vi "Enum from Ring String.vi"(8 "String to Match":string, 9 "Ring Strings []":string[](array[string]), 11 "Ring StringsAndValues[]":T1) -> (0 "error out":errorcluster, 3 "Enum Value":i32)   [LabVIEW 2023]
uses:
  <vilib>/Utility/miscctls.llb/LVStringsAndValuesArrayTypeDef_I32.ctl
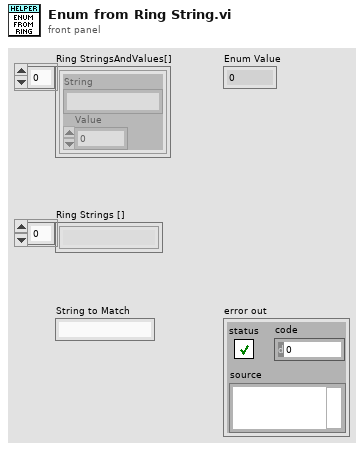
[diagram p1: front panel]
types:
  T1 = typedef "LVStringsAndValuesArrayTypeDef_I32.ctl" = cluster{"String":string, "Value":i32}[]
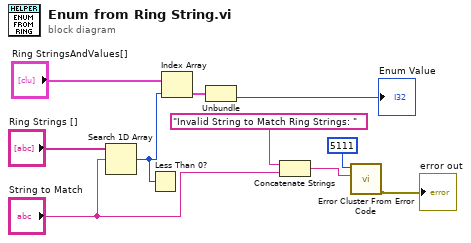
[diagram p0: block diagram]
diagram:
  n1 = Search 1D Array(1D array="Ring Strings []", element="String to Match") -> (index of element=w6:i32)  [unwired: 1 in]
  n2 = Less Than 0?(x=w6) -> ()  [unwired: 1 out]
  n3 = Index Array(array="Ring StringsAndValues[]", index=w6) -> (element=w8:cluster{"String":string, "Value":i32})
  n4 = Unbundle(w8) -> ("Value"=→"Enum Value":i32)  [unwired: 1 out]
  n5 = Concatenate Strings("Invalid String to Match Ring Strings: " ("string"), "String to Match") -> (w1:string)
  n6 = call <vilib>:"Error Cluster From Error Code.vi"("error message (\"\")"=w1, "error code (0)"=5111) -> ("error out"=→"error out":errorcluster)  [unwired: 7 in]
